vi "OverlayRectangle.vi"   [LabVIEW 2024, in "OpenLvVision_Overlays.lvlib"]
doc: "Overlays an recangle on top of the image."
uses:
  OpenLvVision_Overlays.lvlib
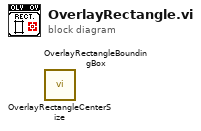
[diagram p0: block diagram]
diagram:
  n1 = call "OverlayRectangleCenterSize.vi"() -> ()  [unwired: 10 in, 2 out]
  n2 = call "OverlayRectangleBoundingBox.vi"() -> ()  [unwired: 10 in, 2 out]
